vi "ProcessHandshakeRequest.vi"(8 "error in (no error)":errorcluster, 10 "HTTP Header":string, 11 "WebSocket in":refnum<class "WebSocket.lvclass">) -> (0 "error out":errorcluster, 1 "Sec-WebSocket-Key":string, 2 "Is Websocket Request?":bool, 3 "WebSocket out":refnum<class "WebSocket.lvclass">, 5 "Host":string)   [LabVIEW 2013, in "WebSockets.lvlib" / "WebSocket.lvclass"]
doc: "Converts the raw HTTP header string into it's main component parts needed to check if the incoming connection is a WS connection. The additional headers are returned in a variant lookup table."
uses:
  WebSocket.lvclass
  WebSocket.lvclass/WebSocket.ctl
  Write Return Headers.vi
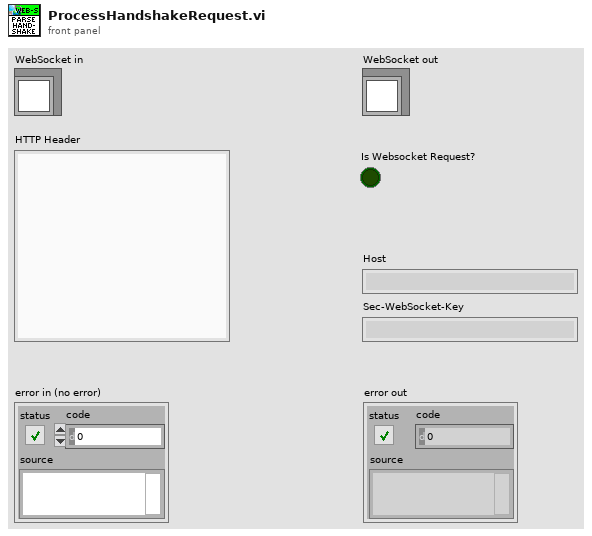
[diagram p1: front panel]
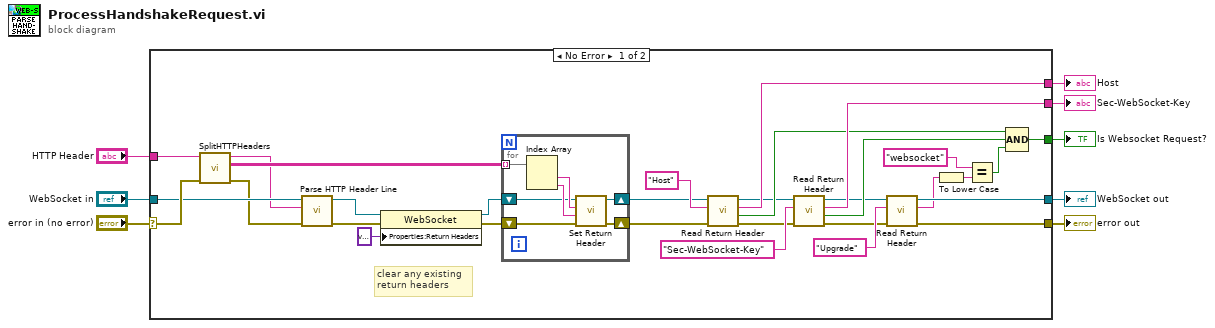
[diagram p0: block diagram]
diagram:
  n1 = case shown="No Error" "error in (no error)" {
    selector: "error in (no error)" -> [w26 w48]
    tunnel: "HTTP Header" -> [w39 _]
    tunnel: [w36 _] -> w7
    tunnel: [w34 _] -> w6
    tunnel: [w31 w47] -> w2
    tunnel: [w27 _] -> w5
    tunnel: [w23 w48] -> w3
    tunnel: "WebSocket in" -> [w13 w47]
    frame No Error {
      # "clear any existing return headers"
      n2 = call "SplitHTTPHeaders.vi"("error in (no error)"=w26, "HTTP Header String"=w39) -> ("error out"=w10:errorcluster, "Headers Array"=w38:string[][], "HTTP Request"=w11:string)  [unwired: 7 in]
      n3 = call-dynamic "Parse HTTP Header Line.vi"("error in (no error)"=w10, "HTTP Header Line"=w11, "WebSocket in"=w13) -> ("error out"=w9:errorcluster, "WebSocket out"=w12:refnum<class "WebSocket.lvclass">)  [unwired: 7 in]
      n4 = property class="WebSocket"(reference=w12, error in=w9, "Properties:Return Headers"=variant ("Return Headers")) -> (reference out=w15:refnum<class "WebSocket.lvclass">, error out=w16:errorcluster)
      n5 = for {
        tunnel: w38 -> [w46] mode=indexing
        shift-right: [w45] -> w17
        shift-left: w15 -> [w40]
        shift-right: [w44] -> w22
        shift-left: w16 -> [w43]
        n6 = Index Array(array=w46) -> (element #1=w42:string, element #2=w41:string)  [unwired: 2 in]
        n7 = call "Set Return Header.vi"("error in (no error)"=w43, "Value"=w41, "Name"=w42, "WebSockets in"=w40) -> ("error out"=w44:errorcluster, "WebSockets out"=w45:refnum<class "WebSocket.lvclass">)  [unwired: 6 in]
      }
      n8 = call "Read Return Header.vi"("error in (no error)"=w22, "Name"="Host" ("name"), "WebSocket in"=w17) -> ("error out"=w25:errorcluster, "Found?"=w33:bool, "Value"=w36:string, "WebSocket out"=w18:refnum<class "WebSocket.lvclass">)  [unwired: 5 in]
      n9 = call "Read Return Header.vi"("error in (no error)"=w25, "Name"="Sec-WebSocket-Key", "WebSocket in"=w18) -> ("error out"=w24:errorcluster, "Found?"=w32:bool, "Value"=w34:string, "WebSocket out"=w19:refnum<class "WebSocket.lvclass">)  [unwired: 5 in]
      n10 = call "Read Return Header.vi"("error in (no error)"=w24, "Name"="Upgrade", "WebSocket in"=w19) -> ("error out"=w23:errorcluster, "Value"=w21:string, "WebSocket out"=w31:refnum<class "WebSocket.lvclass">)  [unwired: 5 in, 1 out]
      n11 = To Lower Case(string=w21) -> (all lower case string=w20:string)
      n12 = Equal?(x="websocket", y=w20) -> (x = y?=w28:bool)
      n13 = Compound Arithmetic op=AND(w33, w32, w28) -> (w27:bool)
    }
    frame Error {
    }
  }
  "Host" <- w7
  "Sec-WebSocket-Key" <- w6
  "Is Websocket Request?" <- w5
  "error out" <- w3
  "WebSocket out" <- w2
